vi "VoltageRatioInputSensorEventExe.vi"(8 "error in (no error)":errorcluster, 10 "Event Registration Refnum In":refnum<event-registration>, 11 "Devices In":u64[](array[numeric])) -> (0 "error out":errorcluster, 1 "Sensor Value":dbl, 2 "Event Registration Refnum Out":refnum<event-registration>, 3 "Devices Out":u64[](array[numeric]), 4 "phid":u64, 5 "Event?":bool, 7 "Index":i32)   [LabVIEW 2012, in "Phidget Voltage Ratio Input.lvlib"]
doc: "${SensorChange:Header}"
uses:
  <instrlib>/Phidgets/Phidget Voltage Ratio Input/Phidget Voltage Ratio Input.lvlib
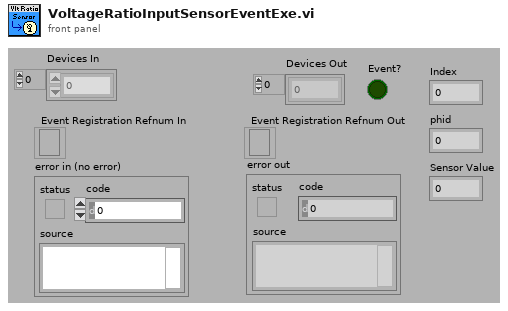
[diagram p1: front panel]
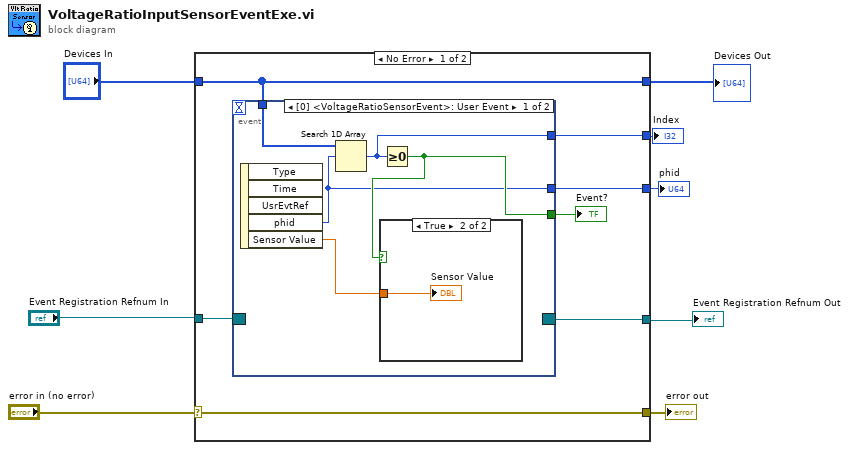
[diagram p0: block diagram]
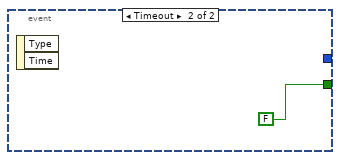
[diagram p3: hidden frame]
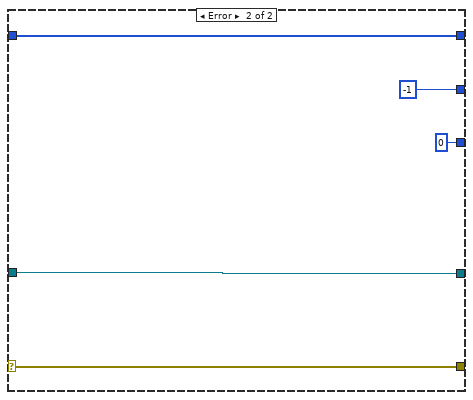
[diagram p4: hidden frame]
diagram:
  n1 = case shown="No Error" "error in (no error)" {
    selector: "error in (no error)" -> [w12 w27]
    tunnel: [w12 w27] -> w7
    tunnel: [w15 w26] -> w1
    tunnel: "Event Registration Refnum In" -> [w14 w26]
    tunnel: [w11 w25] -> w5
    tunnel: "Devices In" -> [w11 w25]
    tunnel: [w10 -1] -> w4
    tunnel: [w9 u64 0 ("phid")] -> w3
    frame No Error {
      n2 = event shown="[0] <VoltageRatioSensorEvent>: User Event" {
        selector: w14 -> [_ _]
        dyn-events: [_ _] -> w15
        timeout: _ -> [_ _]
        tunnel: [w19 FALSE] -> w13
        tunnel: w11 -> [w20 _]
        tunnel: [w18 _] -> w10
        tunnel: [w16 _] -> w9
        event User Event {
          n3 = event-data() -> ("phid"=w16:u64, "Sensor Value"=w17:dbl)  [unwired: 1 in, 3 out]
          n4 = Search 1D Array(1D array=w20, element=w16) -> (index of element=w18:i32)  [unwired: 1 in]
          n5 = Greater Or Equal To 0?(x=w18) -> (x >= 0?=w19:bool)
          n6 = case shown="True" w19 {
            tunnel: w17 -> [_ w21]
            frame False {
            }
            frame True {
              "Sensor Value" <- w21
            }
          }
        }
        event Timeout {
          n7 = event-data() -> ()  [unwired: 1 in, 2 out]
        }
      }
      "Event?" <- w13
    }
    frame Error {
    }
  }
  "error out" <- w7
  "Devices Out" <- w5
  "Index" <- w4
  "phid" <- w3
  "Event Registration Refnum Out" <- w1
